vi "case2.vi"() -> ()   [LabVIEW 2019]
panel:
  out "Numeric 2":i32
  out "Numeric":i32
  out "current time 2":timestamp
  out "current time":timestamp
  in  "stop":bool
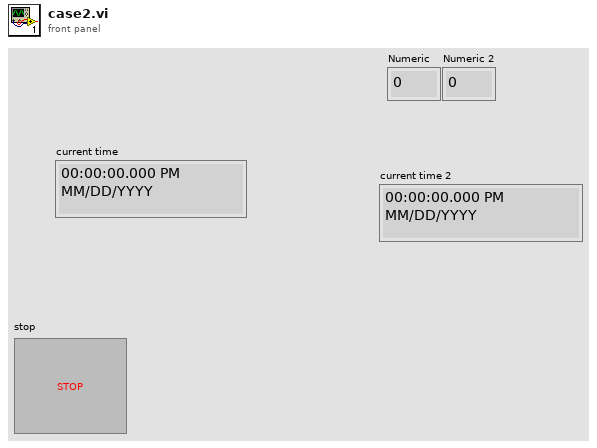
[diagram p1: front panel]
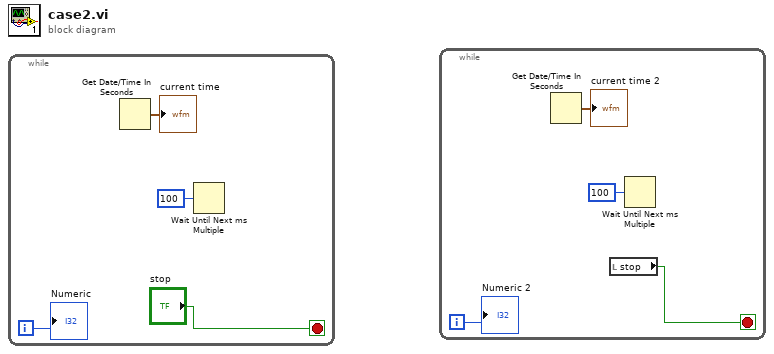
[diagram p0: block diagram]
diagram:
  n1 = while {
    i -> [w2]
    stop <- "stop" stop-if-true
    n2 = Get Date/Time In Seconds() -> (seconds since 1Jan1904=→"current time":timestamp)
    n3 = Wait Until Next ms Multiple(millisecond multiple=u32 100) -> ()  [unwired: 1 out]
    "Numeric" <- w2
  }
  n4 = while {
    i -> [w6]
    stop <- w5 stop-if-true
    n5 = Get Date/Time In Seconds() -> (seconds since 1Jan1904=→"current time 2":timestamp)
    n6 = local read "stop"() -> (w5:bool)
    n7 = Wait Until Next ms Multiple(millisecond multiple=u32 100) -> ()  [unwired: 1 out]
    "Numeric 2" <- w6
  }
